vi "Info.vi"(8 "error in (no error)":errorcluster, 9 "sourceTag":string, 10 "message":string, 11 "Logger in":refnum<class "Logger.lvclass">) -> (0 "error out":errorcluster, 3 "Logger out":refnum<class "Logger.lvclass">)   [LabVIEW 2026, in "Lumberjack.lvlib" / "Logger.lvclass"]
doc: "Logs a message at INFO through the resolved logger.\nConvenience wrapper over Log with the severity fixed to INFO; builds the Statement and hands it to the LogManager for asynchronous fan-out, subject to the global and per-appender thresholds. No-op passthrough if no logger resolves.\nLumberjack.lvlib, Logger.lvclass, public."
uses:
  Logger.lvclass
  TypeDefs/Severity.ctl
  Lumberjack.lvlib
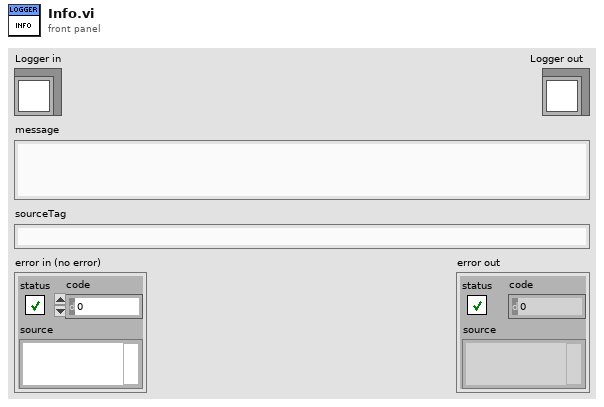
[diagram p1: front panel]
types:
  T1 = typedef "Lumberjack.lvlib/Severity.ctl" = enum16{"OFF", "FATAL", "ERROR", "WARN", "INFO", "DEBUG", "TRACE", "ALL"}
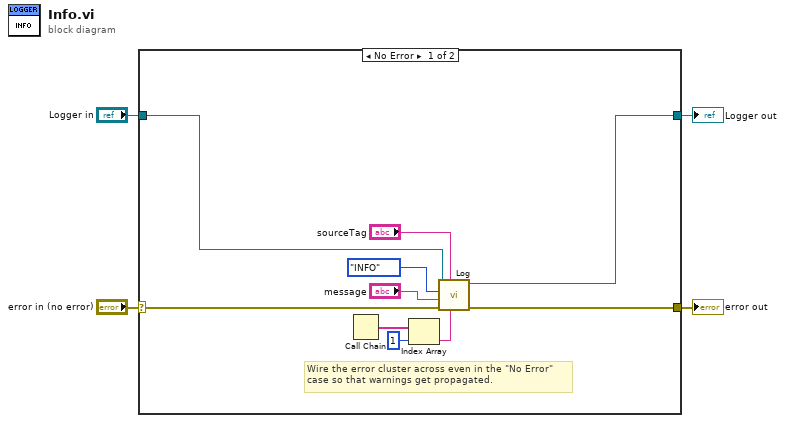
[diagram p0: block diagram]
diagram:
  n1 = case shown="No Error" "error in (no error)" {
    selector: "error in (no error)" -> [w14 w16]
    tunnel: [w5 w16] -> w3
    tunnel: [w9 w15] -> w1
    tunnel: "Logger in" -> [w11 w15]
    frame No Error {
      # "Wire the error cluster across even in the \"No Error\"\ncase so that warnings get propagated."
      n2 = Call Chain() -> (call chain=w8:string[])
      n3 = Index Array(array=w8, index=1) -> (element=w6:string)
      n4 = call "Log.vi"("originVI"=w6, "sourceTag"="sourceTag", "error in (no error)"=w14, "message"="message", "level"=Severity."INFO", "Logger in"=w11) -> ("error out"=w5:errorcluster, "Logger out"=w9:refnum<class "Logger.lvclass">)  [unwired: 4 in]
    }
    frame Error {
    }
  }
  "error out" <- w3
  "Logger out" <- w1
